vi "REM IO - Get IOVar VS refs.vi"(7 "Channel Type":T1, 8 "Fehler (Eingang, kein Fehler)":errorcluster, 9 "Section Name":string, 10 "Item Ref":T2 format="%.0x", 11 "I/O Variable Data in":T3[](array[typedef]) {"VS ref" format="%.0x"}) -> (0 "Fehler (Ausgang)":errorcluster, 2 "Channel Refs":T2[](array[typedef]) format="%.0x", 3 "I/O Variable Data out":T3[](array[typedef]) {"VS ref" format="%.0x"})   [LabVIEW 2019, in "SEECD Engine.lvlib"]
uses:
  SEECD Engine.lvlib
  <vilib>/NI VeriStand/Custom Device API/Custom Device API.lvlib
  Modules.lvlibp/RemIO Module/RemIO Module.lvclass
  <vilib>/NI VeriStand/Custom Device API/Custom Device Item Ref.ctl
  Shared/Type Defs/UDV Data Type.ctl
  Shared/SEECD Shared.lvlib
  <vilib>/NI VeriStand/Custom Device API/Custom Device Channel Type.ctl
  Type Defs/REM IO ECAT Slave IOV Cluster.ctl
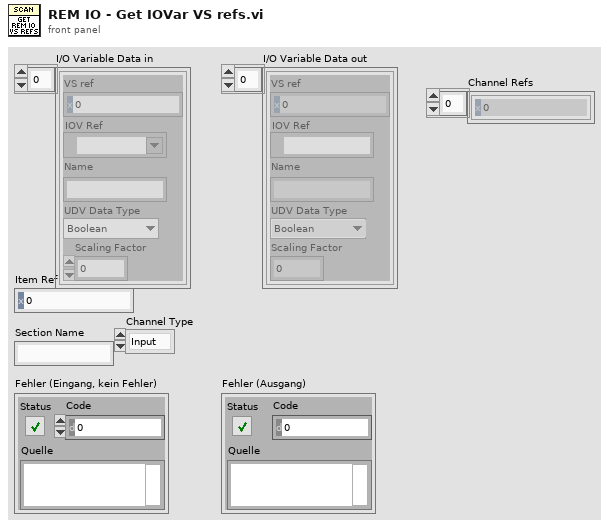
[diagram p1: front panel]
types:
  T1 = typedef "Custom Device API.lvlib/Custom Device Channel Type.ctl" = enum16{"Input", "Output"}
  T2 = typedef "Custom Device API.lvlib/Custom Device Item Ref.ctl" = u64
  T3 = typedef "SEECD Engine.lvlib/REM IO ECAT Slave IOV Cluster.ctl" = cluster{"VS ref":T2, "IOV Ref":refnum<k21>, "Name":string, "UDV Data Type":T4, "Scaling Factor":dbl}
  T4 = typedef "SEECD Shared.lvlib/UDV Data Type.ctl" = enum16{"Boolean", "Fixed Point", "Int8", "Int16", "Int32", "Int64", "U32 Bit Field", "UInt8", "UInt16", "UInt32", "UInt64", "Other", "DBL", "SGL"}
  T5 = typedef "Modules.lvlibp/Custom Device API.lvlib/Custom Device Item Ref.ctl" = u64
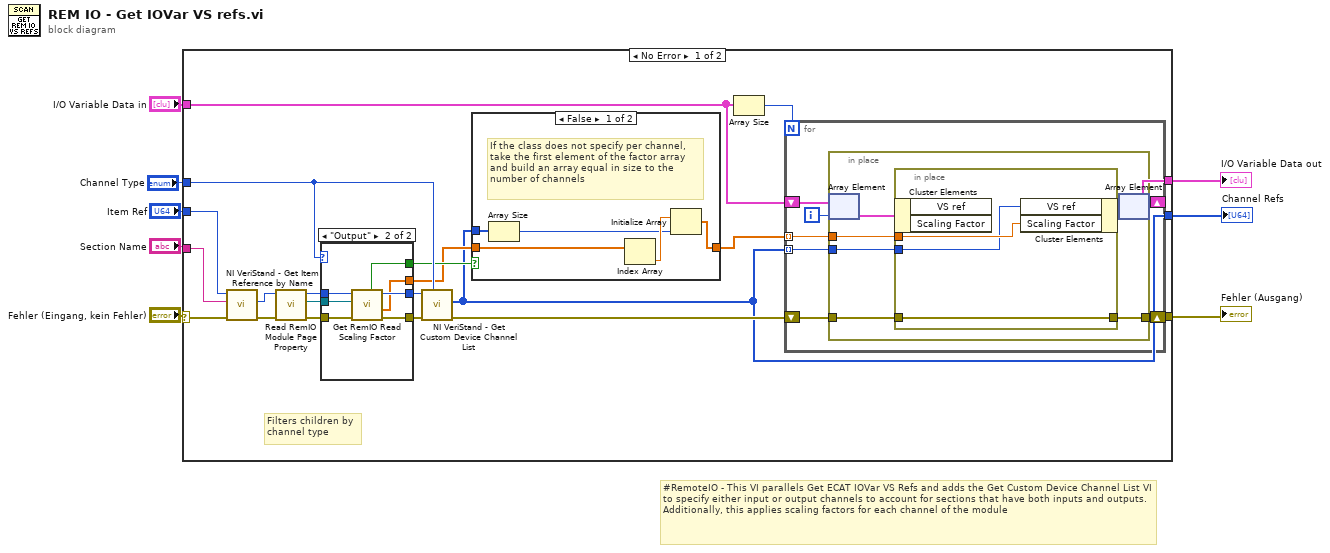
[diagram p0: block diagram]
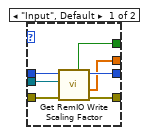
[diagram p3: hidden frame]
diagram:
  # "#RemoteIO - This VI parallels Get ECAT IOVar VS Refs and adds the Get Custom Device Channel List VI to specify either input or output channels to account for sections that have both inputs and outputs.\nAdditionally, this applies scaling factors for each channel of the module"
  n1 = case shown="No Error" "Fehler (Eingang, kein Fehler)" {
    selector: "Fehler (Eingang, kein Fehler)" -> [w23 w66]
    tunnel: "Item Ref" -> [w28 _]
    tunnel: [w25 w65] -> w7
    tunnel: [w27 w66] -> w6
    tunnel: "I/O Variable Data in" -> [w26 w65]
    tunnel: "Section Name" -> [w24 _]
    tunnel: [w10 _] -> w2
    tunnel: "Channel Type" -> [w19 _]
    frame No Error {
      # "Filters children by\nchannel type"
      n2 = call <vilib>:"NI VeriStand - Get Item Reference by Name.vi"("error in (no error)"=w23, "Item Name"=w24, "Parent Ref in"=w28) -> ("error out"=w21:errorcluster, "Item Ref"=w20:T2)  [unwired: 5 in, 2 out]
      n3 = call "Read RemIO Module Page Property.vi"("error in (no error)"=w21, "Node Ptr In"=w20) -> ("error out"=w17:errorcluster, "RemIO Module"=w16:refnum<class "RemIO Module.lvclass">, "Node Ptr Out"=w18:T5)  [unwired: 7 in]
      n4 = case shown="\"Output\"" w19 {
        tunnel: w18 -> [w40 w47]
        tunnel: w17 -> [w41 w48]
        tunnel: [w38 w44] -> w14
        tunnel: [w37 w45] -> w15
        tunnel: [w35 w43] -> w13
        tunnel: [w36 w42] -> w12
        tunnel: w16 -> [w39 w46]
        frame "Input", Default {
          n5 = call-dynamic "Get RemIO Write Scaling Factor.vi"("error in (no error)"=w41, "RemIO Module in"=w39, "Node Ptr In"=w40) -> ("error out"=w37:errorcluster, "Scaling Factors"=w36:dbl[], "Node Ptr Out"=w38:T5, "Per Channel?"=w35:bool)  [unwired: 4 in, 1 out]
        }
        frame "Output" {
          n6 = call-dynamic "Get RemIO Read Scaling Factor.vi"("error in (no error)"=w48, "RemIO Module in"=w46, "Node Ptr In"=w47) -> ("error out"=w45:errorcluster, "Scaling Factors"=w42:dbl[], "Node Ptr Out"=w44:T5, "Per Channel?"=w43:bool)  [unwired: 4 in, 1 out]
        }
      }
      n7 = call <vilib>:"NI VeriStand - Get Custom Device Channel List.vi"("Channel Type"=w19, "error in (no error)"=w15, "Device Ref in"=w14) -> ("error out"=w22:errorcluster, "Specified Channel Ref List"=w10:T2[])  [unwired: 6 in, 1 out]
      n8 = case shown="False" w13 {
        tunnel: w12 -> [w33 w34]
        tunnel: [w31 w34] -> w11
        tunnel: w10 -> [w30 _]
        frame False {
          # "If the class does not specify per channel,\ntake the first element of the factor array\nand build an array equal in size to the\nnumber of channels"
          n9 = Array Size(array=w30) -> (size(s)=w29:i32)
          n10 = Index Array(array=w33) -> (element=w32:dbl)  [unwired: 1 in]
          n11 = Initialize Array(w32, w29) -> (w31:dbl[])
        }
        frame True {
          # "If the class specifies factors by channel,\ndo nothing as the size of the factor array\nwill equal the number of channels"
        }
      }
      n12 = Array Size(array=w26) -> (size(s)=w9:i32)
      n13 = for {
        N: w9 -> [_]
        tunnel: w10 -> [w53] mode=indexing
        shift-right: [w52] -> w25
        shift-left: w26 -> [w55]
        shift-right: [w50] -> w27
        shift-left: w22 -> [w54]
        tunnel: w11 -> [w49] mode=indexing
        i -> [w51]
        n14 = in-place {
          in-place-border: w54 -> [w56]
          in-place-border: w53 -> [w58]
          in-place-border: [w60] -> w50
          in-place-border: w49 -> [w57]
          n15 = in-place-array #1(w55, w51) -> (w59:T3)
          n16 = in-place {
            in-place-border: w58 -> [w62]
            in-place-border: [w64] -> w60
            in-place-border: w56 -> [w64]
            in-place-border: w57 -> [w63]
            n17 = in-place-cluster #2(w59) -> ()  [unwired: 2 out]
            n18 = in-place-cluster #2("VS ref"=w62, "Scaling Factor"=w63) -> (w61:T3)
          }
          n19 = in-place-array #1(w61) -> (w52:T3[])  [unwired: 1 out]
        }
      }
    }
    frame Error {
    }
  }
  "I/O Variable Data out" <- w7
  "Fehler (Ausgang)" <- w6
  "Channel Refs" <- w2
